vi "V-Meter Test Communications.vi"(8 "error in (no error)":errorcluster, 11 "VISA resource name in":refnum<visa-resource-name>) -> (0 "error out":errorcluster, 3 "VISA resource name out":refnum<visa-resource-name>)   [LabVIEW 2016, in "Hall Effect Library.lvlib"]
uses:
  Hall Effect Library.lvlib
  Global Variables/Instruments.vi
  V-Meter Test Communications (2000).vi
  V-Meter Test Communications (2182A).vi
  V-Meter Test Communications (3706).vi
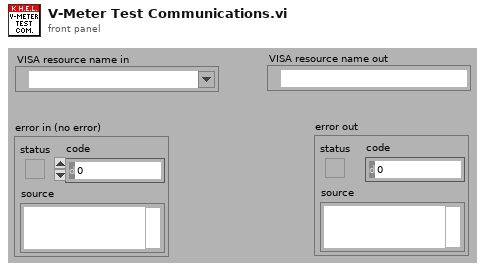
[diagram p1: front panel]
types:
  T1 = typedef "Hall Effect Library.lvlib/Voltmeters.ctl" = enum16{"2000", "2182A", "3706A"}
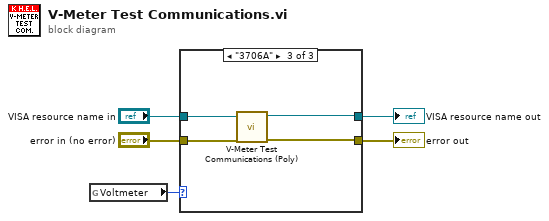
[diagram p0: block diagram]
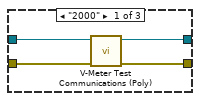
[diagram p2: hidden frame]
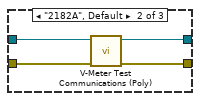
[diagram p3: hidden frame]
diagram:
  n1 = global read "Instruments.vi" "Voltmeter"() -> (w5:T1)
  n2 = case shown="\"3706A\"" w5 {
    tunnel: "error in (no error)" -> [w9 w13 w16]
    tunnel: [w8 w12 w14] -> w1
    tunnel: [w7 w11 w15] -> w2
    tunnel: "VISA resource name in" -> [w6 w10 w17]
    frame "2000" {
      n3 = call-poly "V-Meter Test Communications (Poly).vi"("error in (no error)"=w9, "VISA resource name in"=w6) -> ("error out"=w8:errorcluster, "VISA resource name out"=w7:refnum<visa-resource-name>)  [unwired: 8 out]
    }
    frame "2182A", Default {
      n4 = call-poly "V-Meter Test Communications (Poly).vi"("error in (no error)"=w13, "VISA resource name in"=w10) -> ("error out"=w12:errorcluster, "VISA resource name out"=w11:refnum<visa-resource-name>)  [unwired: 8 out]
    }
    frame "3706A" {
      n5 = call-poly "V-Meter Test Communications (Poly).vi"("error in (no error)"=w16, "VISA resource name in"=w17) -> ("error out"=w14:errorcluster, "VISA resource name out"=w15:refnum<visa-resource-name>)  [unwired: 8 in]
    }
  }
  "error out" <- w1
  "VISA resource name out" <- w2
